vi "Design Challenge _ HW2 V1.vi"() -> ()   [LabVIEW 2025]
panel:
  out "XY Graph":cluster{"Y":dbl[], "Y":dbl[]}[](graph)
  out "X":dbl
  out "Height - Y":dbl
  in  "Initial Height":dbl
  in  "Alpha":dbl
  in  "Initial Velocity":dbl
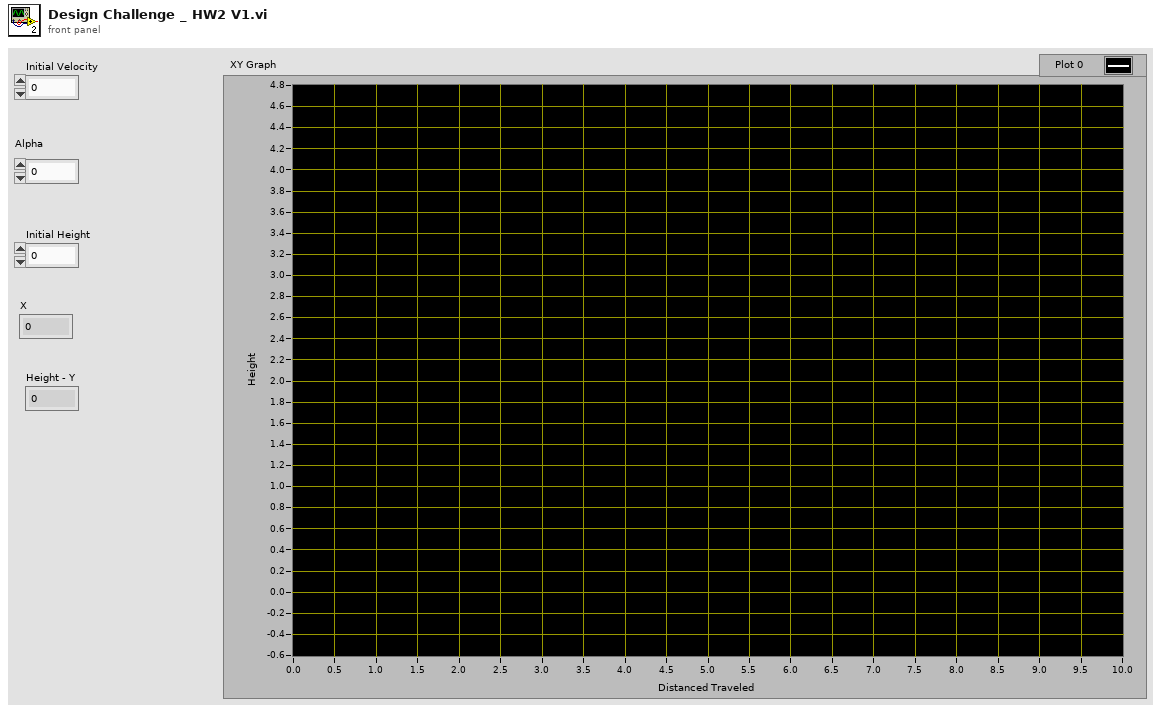
[diagram p1: front panel]
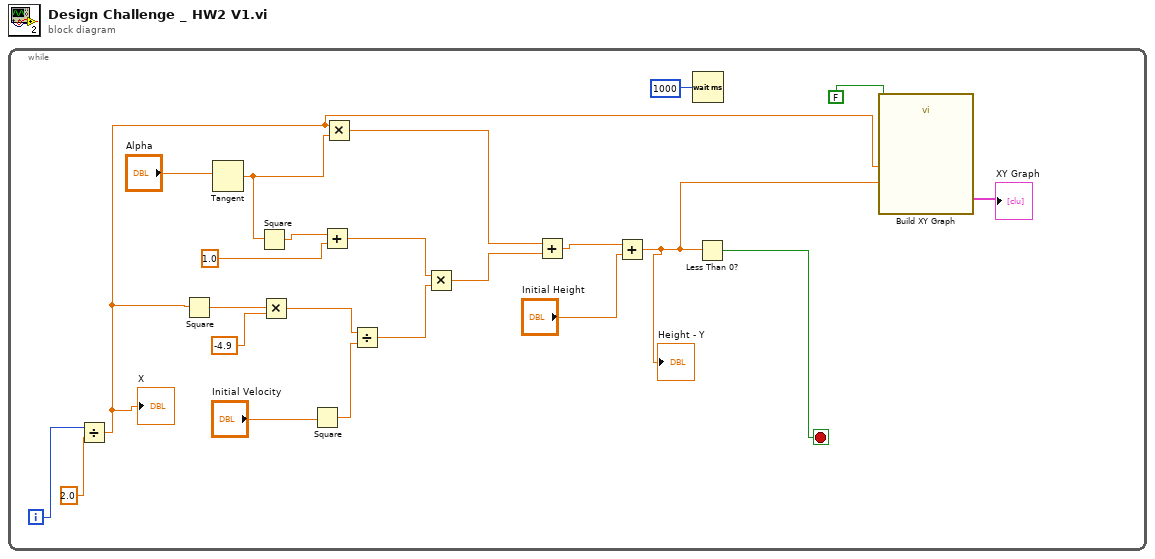
[diagram p0: block diagram]
diagram:
  n1 = while {
    i -> [w22]
    stop <- w6 stop-if-true
    n2 = Divide(x=w22, y=2.0) -> (x/y=w4:dbl)
    "X" <- w4
    n3 = Square(x=w4) -> (x^2=w17:dbl)
    n4 = Tangent(1:"Alpha") -> (0:w20:dbl)
    n5 = Square(x=w20) -> (x^2=w18:dbl)
    n6 = Multiply(x=w17, y=-4.9) -> (x*y=w14:dbl)
    n7 = Square(x="Initial Velocity") -> (x^2=w13:dbl)
    n8 = Add(x=w18, y=1.0) -> (x+y=w12:dbl)
    n9 = Multiply(x=w4, y=w20) -> (x*y=w10:dbl)
    n10 = Divide(x=w14, y=w13) -> (x/y=w11:dbl)
    n11 = Multiply(x=w12, y=w11) -> (x*y=w9:dbl)
    n12 = Add(x=w10, y=w9) -> (x+y=w7:dbl)
    n13 = Add(x=w7, y="Initial Height") -> (x+y=w3:dbl)
    "Height - Y" <- w3
    n14 = Wait (ms)(milliseconds to wait=u32 1000 ("millisecond timer value")) -> ()  [unwired: 1 out]
    n15 = Less Than 0?(x=w3) -> (x < 0?=w6:bool)
    n16 = call "Build XY Graph"("Reset"=FALSE, "Y Input"=w3, "X Input"=w4) -> ("XY Graph"=→"XY Graph":cluster{"X":dbl[], "Y":dbl[]}[])  [unwired: 7 in, 1 out]
  }
